vi "Score and Sort Objects.vi"(7 "Targets":i32=3, 11 "Object Info":T2(array[cluster])) -> (3 "Object Info":T1(array[cluster]))   [LabVIEW 2025]
doc: "Calculate normalized scores and rank based on how well the particles are described by a circle."
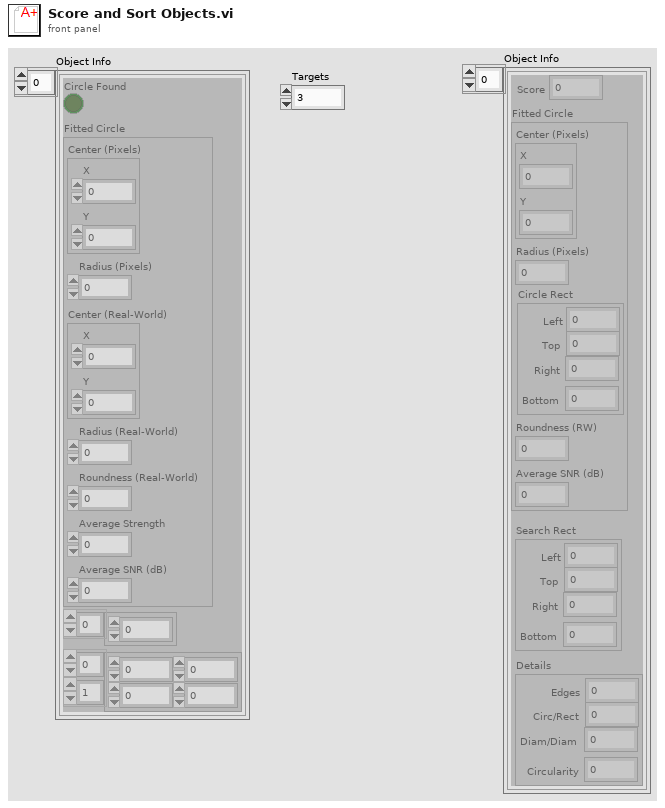
[diagram p1: front panel]
types:
  T1 = cluster{"Score":dbl, "Fitted Circle":cluster{"Center (Pixels)":cluster{"X":sgl, "Y":sgl}, "Radius (Pixels)":dbl, "Circle Rect":cluster{"Left":sgl, "Top":sgl, "Right":sgl, "Bottom":sgl}, "Roundness (RW)":dbl, "Average SNR (dB)":dbl}, "Search Rect":cluster{"Left":sgl, "Top":sgl, "Right":sgl, "Bottom":sgl}, "Details":cluster{"Edges":sgl, "Circ/Rect":sgl, "Diam/Diam":sgl, "Circularity":sgl}}[]
  T2 = cluster{"Circle Found":bool, "Fitted Circle":cluster{"Center (Pixels)":cluster{"X":sgl, "Y":sgl}, "Radius (Pixels)":dbl, "Center (Real-World)":cluster{"X":sgl, "Y":sgl}, "Radius (Real-World)":dbl, "Roundness (Real-World)":dbl, "Average Strength":dbl, "Average SNR (dB)":dbl}, dbl[], dbl[][]}[]
  T3 = cluster{"Bottom":sgl, "Fitted Circle":cluster{"Center (Pixels)":cluster{"X":sgl, "Y":sgl}, "Radius (Pixels)":dbl, "Rect":cluster{"Left":sgl, "Top":sgl, "Right":sgl, "Bottom":sgl}, "Roundness (RW)":dbl, "Average SNR (dB)":dbl}, "Rect":cluster{"Left":sgl, "Top":sgl, "Right":sgl, "Bottom":sgl}, "Rect 2":cluster{"Left":sgl, "Top":sgl, "Right":sgl, "Bottom":sgl}}[]
  T4 = cluster{"Center (Pixels)":cluster{"X":sgl, "Y":sgl}, "Radius (Pixels)":dbl, "Center (Real-World)":cluster{"X":sgl, "Y":sgl}, "Radius (Real-World)":dbl, "Roundness (Real-World)":dbl, "Average Strength":dbl, "Average SNR (dB)":dbl}
  T5 = cluster{"[0]":dbl, "[1]":dbl, "[2]":dbl, "[3]":dbl}
  T6 = cluster{cluster{dbl, dbl}, "Radius (Pixels)":dbl, cluster{dbl, dbl, dbl, dbl}, "Roundness (Real-World)":dbl, "Average SNR (dB)":dbl}
  T7 = cluster{"Score":dbl, "Score":dbl, "Score out":dbl, "Score out":dbl}
  T8 = cluster{dbl, cluster{cluster{dbl, dbl}, "Radius (Pixels)":dbl, cluster{dbl, dbl, dbl, dbl}, "Roundness (Real-World)":dbl, "Average SNR (dB)":dbl}, cluster{"[0]":dbl, "[1]":dbl, "[2]":dbl, "[3]":dbl}, cluster{"Score":dbl, "Score":dbl, "Score out":dbl, "Score out":dbl}}
  T9 = cluster{"Bottom":dbl, "Fitted Circle":cluster{"Center (Pixels)":cluster{"X":dbl, "Y":dbl}, "Radius (Pixels)":dbl, "Rect":cluster{"Left":dbl, "Top":dbl, "Right":dbl, "Bottom":dbl}, "Roundness (Real-World)":dbl, "Average SNR (dB)":dbl}, "Rect":cluster{"[0]":dbl, "[1]":dbl, "[2]":dbl, "[3]":dbl}, "Rect 2":cluster{"Score":dbl, "Score":dbl, "Score out":dbl, "Score out":dbl}}[]
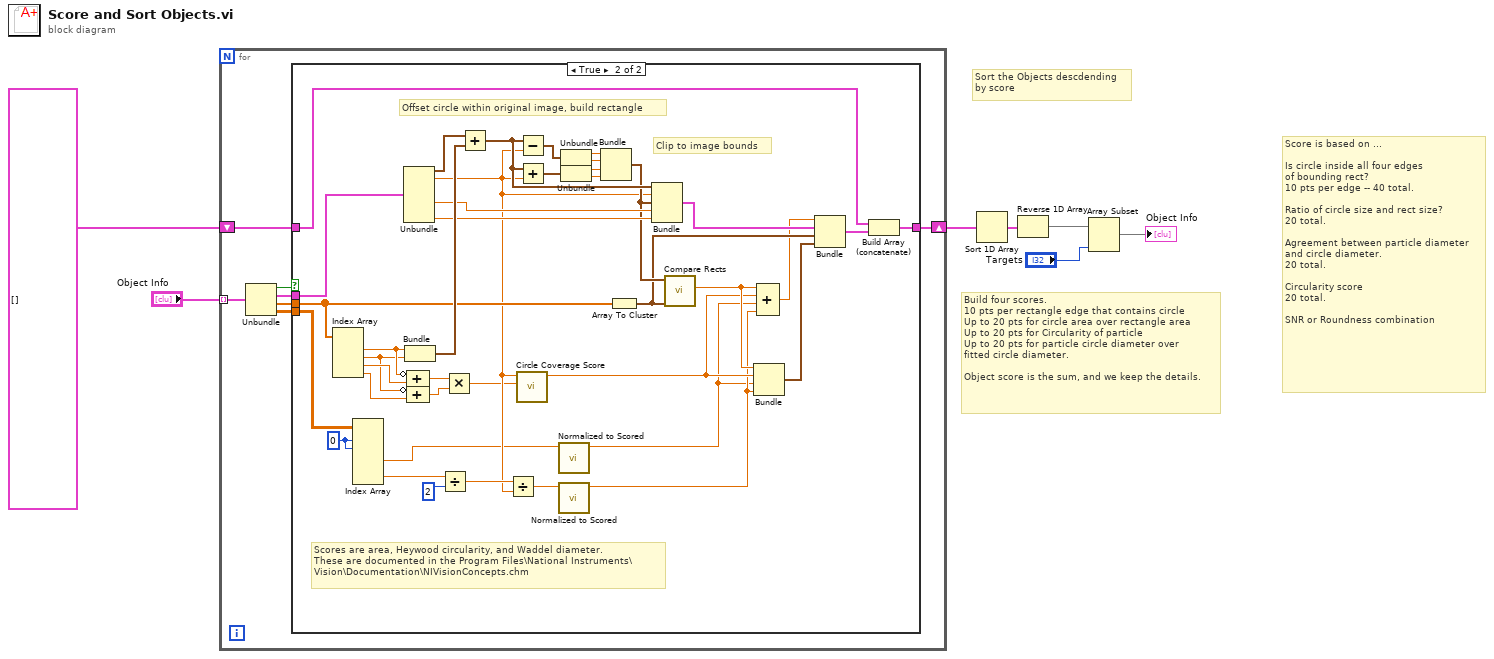
[diagram p0: block diagram]
diagram:
  # "Build four scores.\n10 pts per rectangle edge that contains circle\nUp to 20 pts for circle area over rectangle area\nUp to 20 pts for Circularity of particle\nUp to 20 pts for particle circle diameter over\nfitted circle diameter.\n\nObject score is the sum, and we keep the details."
  # "Sort the Objects descdending\nby score"
  # "Score is based on ...\n\nIs circle inside all four edges\nof bounding rect?\n10 pts per edge -- 40 total.\n\nRatio of circle size and rect size?\n20 total.\n\nAgreement between particle diameter\nand circle diameter.\n20 total.\n\nCircularity score\n20 total.\n\nSNR or Roundness combination"
  n1 = for {
    tunnel: "Object Info" -> [w10] mode=indexing
    shift-right: [w9] -> w5
    shift-left: T3 [] ("Object Info 2") -> [w8]
    n2 = Unbundle(w10) -> ("Circle Found"=w11:bool, "Fitted Circle"=w14:T4, w13:dbl[], w12:dbl[][])
    n3 = case shown="True" w11 {
      tunnel: w14 -> [_ w38]
      tunnel: w13 -> [_ w31]
      tunnel: w12 -> [_ w35]
      tunnel: [w15 w32] -> w9
      tunnel: w8 -> [w15 w34]
      frame False {
      }
      frame True {
        w50 = 0 ("index (row)")
        # "Clip to image bounds"
        # "Scores are area, Heywood circularity, and Waddel diameter.\nThese are documented in the Program Files\\National Instruments\\\nVision\\Documentation\\NIVisionConcepts.chm"
        # "Offset circle within original image, build rectangle"
        n4 = Index Array(array=w31) -> (element #1=w54:dbl, element #2=w52:dbl, element #3=w53:dbl, element #4=w51:dbl)  [unwired: 4 in]
        n5 = Index Array(array=w35, index (row) #1=w50, index (col) #1=w50) -> (element #2=w17:dbl, element #3=w49:dbl)  [unwired: 4 in, 1 out]
        n6 = Unbundle(w38) -> ("Center (Pixels)"=w39:cluster{"X":sgl, "Y":sgl}, "Radius (Pixels)"=w26:dbl, "Roundness (Real-World)"=w37:dbl, "Average SNR (dB)"=w36:dbl)  [unwired: 3 out]
        n7 = Bundle("Numeric"=w54, "Numeric"=w52) -> (w55:cluster{"Numeric":dbl, "Numeric":dbl})  [unwired: 1 in]
        n8 = Compound Arithmetic op=ADD(invert w54, w53) -> (w25:dbl)
        n9 = Compound Arithmetic op=ADD(invert w52, w51) -> (w24:dbl)
        n10 = Divide(x=w49, y=2 ("index (row)")) -> (x/y=w47:dbl)
        n11 = Multiply(x=w25, y=w24) -> (x*y=w23:dbl)
        n12 = Add(x=w39, y=w55) -> (x+y=w30:cluster{dbl, dbl})
        n13 = Divide(x=w47, y=w26) -> (x/y=w21:dbl)
        n14 = call "Circle Coverage Score.vi"("Rect Area"=w23, "Radius"=w26) -> ("Score"=w22:dbl)  [unwired: 9 in]
        n15 = Subtract(x=w30, y=w26) -> (x-y=w40:cluster{dbl, dbl})
        n16 = Add(x=w30, y=w26) -> (x+y=w41:cluster{dbl, dbl})
        n17 = call "Normalized to Scored.vi"("Normalized in"=w17) -> ("Score out"=w16:dbl)  [unwired: 10 in]
        n18 = call "Normalized to Scored.vi"("Normalized in"=w21) -> ("Score out"=w20:dbl)  [unwired: 10 in]
        n19 = Unbundle(w40) -> (w45:dbl, w44:dbl)
        n20 = Unbundle(w41) -> (w43:dbl, w42:dbl)
        n21 = Bundle(w45, w44, w43, w42) -> (w29:cluster{dbl, dbl, dbl, dbl})  [unwired: 1 in]
        n22 = Array To Cluster(array=w31) -> (cluster=w27:T5)
        n23 = Bundle(w30, "Radius (Pixels)"=w26, w29, "Roundness (Real-World)"=w37, "Average SNR (dB)"=w36) -> (w46:T6)  [unwired: 1 in]
        n24 = call "Compare Rects.vi"("Bounding Rect"=w27, "Circle Rect"=w29) -> ("Score"=w28:dbl)  [unwired: 9 in]
        n25 = Bundle("Score"=w28, "Score"=w22, "Score out"=w16, "Score out"=w20) -> (w18:T7)  [unwired: 1 in]
        n26 = Compound Arithmetic op=ADD(w28, w22, w16, w20) -> (w19:dbl)
        n27 = Bundle(w19, w46, w27, w18) -> (w33:T8)  [unwired: 1 in]
        n28 = Build Array (concatenate)(w34, w33) -> (w32:T9)
      }
    }
  }
  n29 = Sort 1D Array(array=w5) -> (sorted array=w4:T9)
  n30 = Reverse 1D Array(array=w4) -> (reversed array=w3:T9)
  n31 = Array Subset(array=w3, length="Targets") -> (→"Object Info":T9)  [unwired: 1 in]
